vi "Distance PWM-Close.vi"(8 "Error":errorcluster, 11 "SonarMB1010DigitalDevRef":T1={"CounterDevRef"={"DevStatus"={"status"=FALSE, "code"=0, "source"=""}, "CntIndex"=enum."Invalid"}, "Min Distance"=0.000147, "Max Distance"=0.000147, "PWM Frequency"=0.0, "DIO Channel"=enum."DIO 0"}) -> (0 "Error Out":errorcluster)   [LabVIEW 2017]
doc: "Closes the reference to the ultrasonic sensor you specify. Use this VI to close each ultrasonic sensor reference that you open with the Open VI.\n\nThis software is licensed. Open the labview\\readme\\WPI Robotics Library Open Source License.txt file for more information."
uses:
  TypeDefs Distance/Cluster_Distance PWM Reference.ctl
  <vilib>/Rock Robotics/WPI/Counter/WPI_CounterDevRef.ctl
  <vilib>/Rock Robotics/SystemInterfaces/Counter/FPGA_CounterCtrSystemIndex.ctl
  <vilib>/Rock Robotics/SystemInterfaces/DIO/FPGA_DIOChannel.ctl
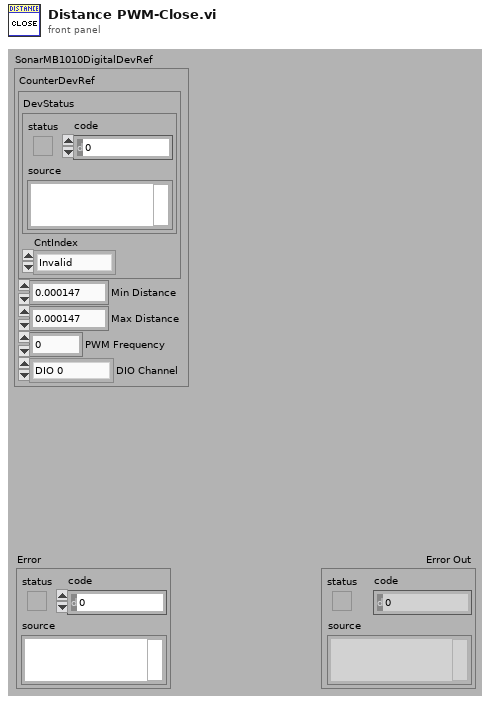
[diagram p1: front panel]
types:
  T1 = typedef "Cluster_Distance PWM Reference.ctl" = cluster{"CounterDevRef":T2, "Min Distance":dbl, "Max Distance":dbl, "PWM Frequency":dbl, "DIO Channel":T4}
  T2 = typedef "WPI_CounterDevRef.ctl" = cluster{"DevStatus":errorcluster, "CntIndex":T3}
  T3 = typedef "FPGA_CounterCtrSystemIndex.ctl" = enum8{"Ctr 0", "Ctr 1", "Ctr 2", "Ctr 3", "Ctr 4", "Ctr 5", "Ctr 6", "Ctr 7", "Invalid"}
  T4 = typedef "FPGA_DIOChannel.ctl" = enum8{"DIO 0", "DIO 1", "DIO 2", "DIO 3", "DIO 4", "DIO 5", "DIO 6", "DIO 7", "DIO 8", "DIO 9", "DIO MXP 0", "DIO MXP 1", "DIO MXP 2", "DIO MXP 3", "DIO MXP 4", "DIO MXP 5", "DIO MXP 6", "DIO MXP 7", "DIO MXP 8", "DIO MXP 9", "DIO MXP 10", "DIO MXP 11", "DIO MXP 12", "DIO MXP 13", "DIO MXP 14", "DIO MXP 15", "SPI Port CS1", "SPI Port CS2", "SPI Port CS3", "SPI Port MISO", "SPI Port MOSI", "Invalid"}
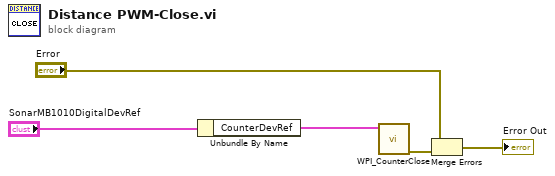
[diagram p0: block diagram]
diagram:
  n1 = Unbundle By Name("SonarMB1010DigitalDevRef") -> ("CounterDevRef"=w1:T2)
  n2 = call <vilib>:"WPI_CounterClose.vi"("CounterDevRef"=w1) -> ("error out"=w4:errorcluster)  [unwired: 10 in]
  n3 = Merge Errors("Error", w4) -> (→"Error Out":errorcluster)
